vi "Player Bar Example.vi"() -> ()   [LabVIEW 2016]
panel:
  out "Image 2":T1(plugin-control)
  in  "stop":bool
  out "Image":T1(plugin-control)
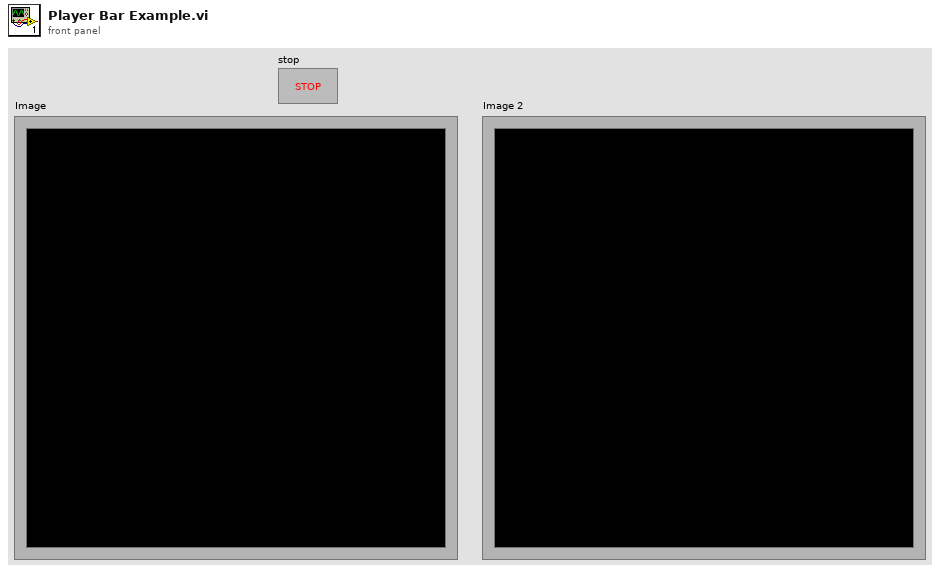
[diagram p1: front panel]
types:
  T1 = typedef "IMAQ Image.ctl" = refnum<image>
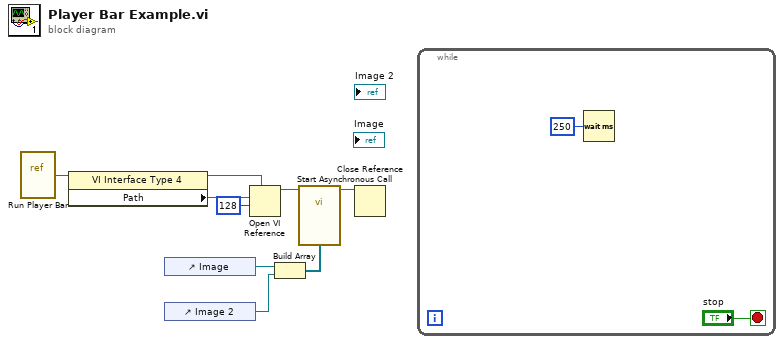
[diagram p0: block diagram]
diagram:
  n1 = vi-ref "Run Player Bar.vi"() -> (w5:refnum<vi>)
  n2 = property class="VI Interface Type 4"(reference=w5) -> (reference out=w9:refnum<vi>, "Path"=w6:path)  [unwired: 1 in, 1 out]
  n3 = control-ref of="Image"() -> (w3:refnum<vi>)
  n4 = control-ref of="Image 2"() -> (w1:refnum<vi>)
  n5 = Open VI Reference(type specifier VI Refnum (for type only)=w9, vi path=w6, options=128) -> (vi reference=w4:refnum<vi>)  [unwired: 3 in, 1 out]
  n6 = Build Array(w3, w1) -> (w2:refnum<vi>[])
  n7 = call-by-ref "Start Asynchronous Call"(reference=w4, "IMAQ Display Refs"=w2) -> (reference out=w8:refnum<vi>)  [unwired: 16 in, 1 out]
  n8 = Close Reference(reference=w8) -> ()  [unwired: 1 in, 1 out]
  n9 = while {
    stop <- "stop" stop-if-true
    n10 = Wait (ms)(milliseconds to wait=u32 250) -> ()  [unwired: 1 out]
  }
